vi "graph & save averages.vi"() -> ()   [LabVIEW 2018]
uses:
  <vilib>/Waveform/WDTOps.llb/WDT Append Waveforms DBL.vi
panel:
  in  "Polarimeter":path=path "C:/Users/severinm/Desktop/other diode.lvm"
  in  "Germanium":path=path "C:/Users/severinm/Desktop/germaniam diode.lvm"
  out "Waveform Graph 2":waveform(dbl)(graph)
  out "Waveform Graph":waveform(dbl)(graph)
  in  "stop":bool
  in  "Write Averages?":bool
  in  "Which power of 10?":dbl min=1.0 step=1.0
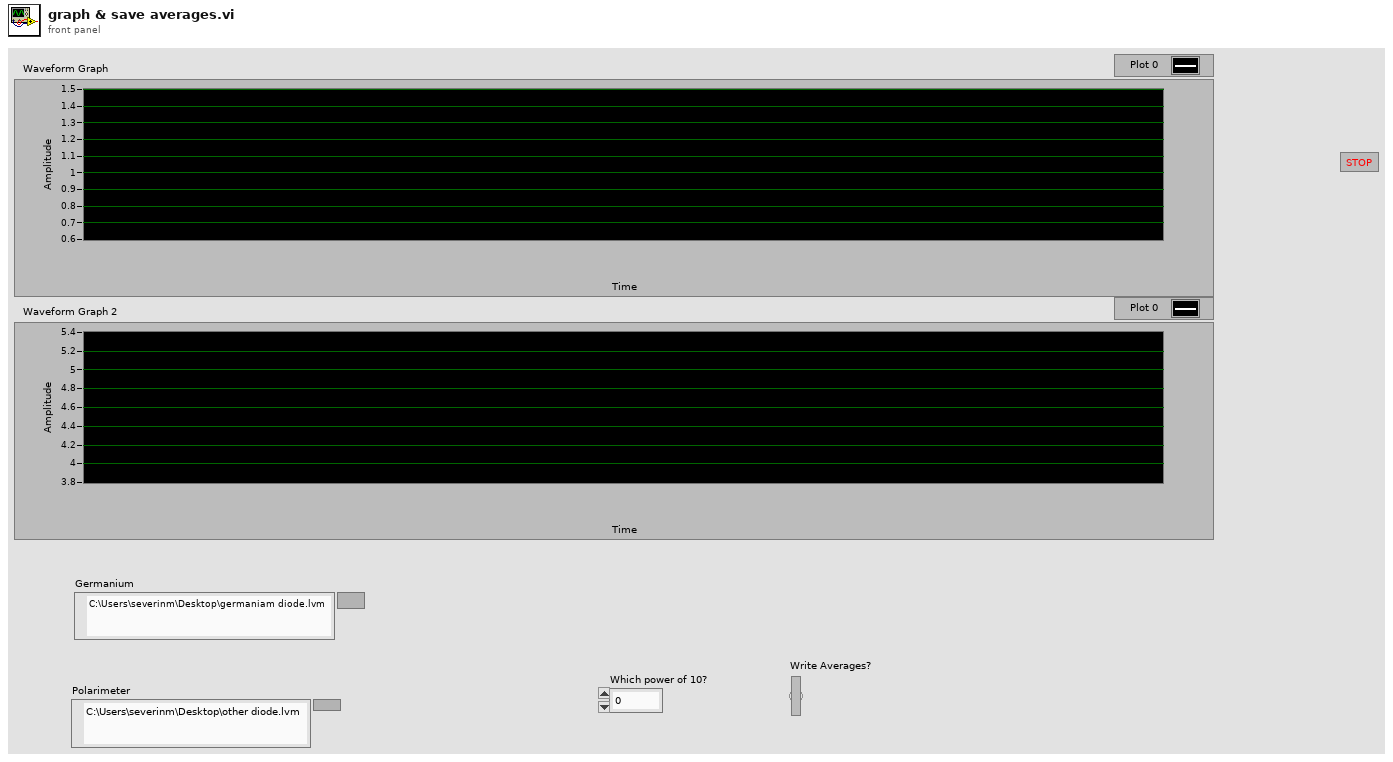
[diagram p1: front panel]
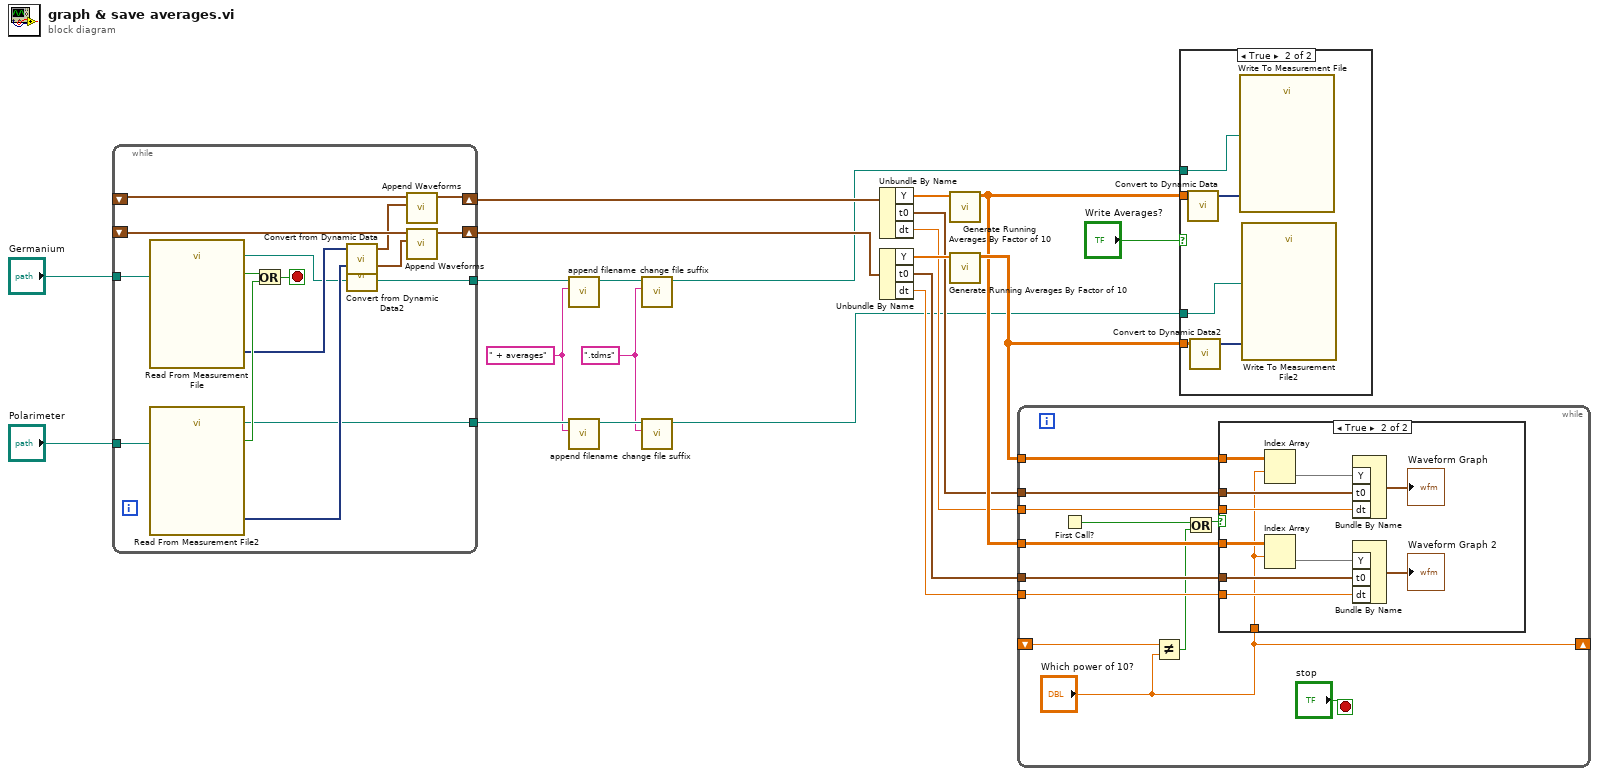
[diagram p0: block diagram]
diagram:
  w1 = ".tdms" ("string")
  w4 = " + averages" ("string")
  n1 = while {
    shift-right: [w33] -> w21
    shift-left: _ -> [w31]
    shift-right: [w32] -> w18
    shift-left: _ -> [w30]
    tunnel: "Polarimeter" -> [w25]
    tunnel: "Germanium" -> [w24]
    tunnel: [w23] -> w8
    tunnel: [w22] -> w6
    stop <- w35 stop-if-true
    n2 = call "Read From Measurement File"("Filename"=w24) -> ("Filename Out"=w22:path, "Signals"=w26:dynamicdata, "EOF?"=w36:bool)  [unwired: 5 in, 3 out]
    n3 = call "Read From Measurement File2"("Filename"=w25) -> ("Filename Out"=w23:path, "Signals"=w27:dynamicdata, "EOF?"=w34:bool)  [unwired: 5 in, 3 out]
    n4 = Or(x=w36, y=w34) -> (x .or. y?=w35:bool)
    n5 = call "Convert from Dynamic Data"("Dynamic Data Type"=w26) -> ("Waveform"=w29:waveform(dbl))  [unwired: 3 in]
    n6 = call "Convert from Dynamic Data2"("Dynamic Data Type"=w27) -> ("Waveform"=w28:waveform(dbl))  [unwired: 3 in]
    n7 = call-poly <vilib>:"Append Waveforms.vi"("waveform B"=w29, "waveform A"=w31) -> ("waveform out"=w33:waveform(dbl))  [unwired: 8 in, 1 out]
    n8 = call-poly <vilib>:"Append Waveforms.vi"("waveform B"=w28, "waveform A"=w30) -> ("waveform out"=w32:waveform(dbl))  [unwired: 8 in, 1 out]
  }
  n9 = call "append filename.vi"("string"=w4, "path"=w6) -> ("path 2"=w5:path)  [unwired: 9 in]
  n10 = call "append filename.vi"("string"=w4, "path"=w8) -> ("path 2"=w7:path)  [unwired: 9 in]
  n11 = call "change file suffix.vi"("new suffix"=w1, "path"=w5) -> ("path 2"=w3:path)  [unwired: 9 in]
  n12 = call "change file suffix.vi"("new suffix"=w1, "path"=w7) -> ("path 2"=w2:path)  [unwired: 9 in]
  n13 = Unbundle By Name(w21) -> ("Y"=w20:dbl[], "t0"=w14:timestamp, "dt"=w13:dbl)
  n14 = Unbundle By Name(w18) -> ("Y"=w19:dbl[], "t0"=w12:timestamp, "dt"=w11:dbl)
  n15 = call "Generate Running Averages By Factor of 10.vi"("Input"=w20) -> ("Averages"=w16:dbl[][])  [unwired: 10 in]
  n16 = call "Generate Running Averages By Factor of 10.vi"("Input"=w19) -> ("Averages"=w17:dbl[][])  [unwired: 10 in]
  n17 = while {
    tunnel: w17 -> [w47]
    tunnel: w16 -> [w46]
    tunnel: w14 -> [w45]
    tunnel: w13 -> [w44]
    tunnel: w12 -> [w43]
    tunnel: w11 -> [w42]
    shift-right: ["Which power of 10?"] -> _
    shift-left: _ -> [w40]
    stop <- "stop" stop-if-true
    n18 = First Call?() -> (First Call?: T/F=w41:bool)
    n19 = Not Equal?(x=w40, y="Which power of 10?") -> (x != y?=w37:bool)
    n20 = Or(x=w41, y=w37) -> (x .or. y?=w38:bool)
    n21 = case shown="True" w38 {
      tunnel: w47 -> [_ w59]
      tunnel: w46 -> [_ w58]
      tunnel: "Which power of 10?" -> [_ w49]
      tunnel: w45 -> [_ w55]
      tunnel: w44 -> [_ w54]
      tunnel: w43 -> [_ w53]
      tunnel: w42 -> [_ w52]
      frame False {
      }
      frame True {
        n22 = Index Array(array=w59, index (row)=w49) -> (element=w57:dbl[])  [unwired: 1 in]
        n23 = Index Array(array=w58, index (row)=w49) -> (element=w56:dbl[])  [unwired: 1 in]
        n24 = Bundle By Name("Y"=w57, "t0"=w55, "dt"=w54) -> (→"Waveform Graph":waveform(dbl))  [unwired: 1 in]
        n25 = Bundle By Name("Y"=w56, "t0"=w53, "dt"=w52) -> (→"Waveform Graph 2":waveform(dbl))  [unwired: 1 in]
      }
    }
  }
  n26 = case shown="True" "Write Averages?" {
    tunnel: w3 -> [_ w64]
    tunnel: w2 -> [_ w62]
    tunnel: w17 -> [_ w61]
    tunnel: w16 -> [_ w60]
    frame False {
    }
    frame True {
      n27 = call "Convert to Dynamic Data"("2D Array"=w60) -> ("Dynamic Data Type"=w65:dynamicdata)  [unwired: 3 in]
      n28 = call "Convert to Dynamic Data2"("2D Array"=w61) -> ("Dynamic Data Type"=w63:dynamicdata)  [unwired: 3 in]
      n29 = call "Write To Measurement File"("Signals"=w65, "Filename"=w64) -> ()  [unwired: 15 in, 3 out]
      n30 = call "Write To Measurement File2"("Signals"=w63, "Filename"=w62) -> ()  [unwired: 15 in, 3 out]
    }
  }
